vi "Get Teams.vi"(6 "Authorization":T2[](array[typedef]), 8 "error in (no error)":errorcluster) -> (0 "error out":errorcluster, 3 "Teams Out":T1(array[cluster]))   [LabVIEW 2016]
uses:
  <vilib>/addons/_JKI.lib/REST Client/classes/REST Client/HTTP Header.ctl
  <vilib>/addons/_JKI.lib/REST Client/classes/REST Client/REST Client.lvclass
  <vilib>/addons/_JKI.lib/Serialization/JSON/JKI JSON Serialization.lvlib
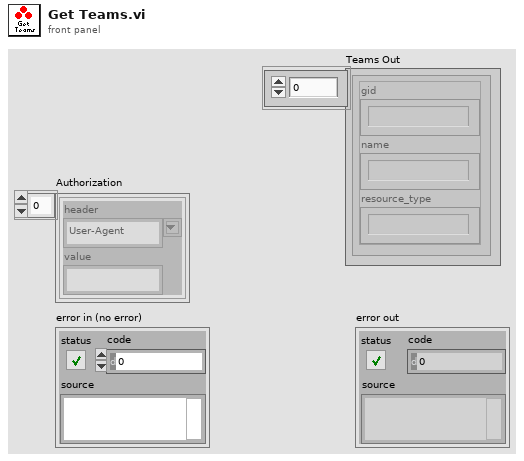
[diagram p1: front panel]
types:
  T1 = cluster{"gid":string, "name":string, "resource_type":string}[]
  T2 = typedef "REST Client.lvlib/REST Client.lvclass/HTTP Header.ctl" = cluster{"header":string, "value":string}
  T3 = cluster{"data":cluster{"gid":string, "name":string, "resource_type":string}[]}
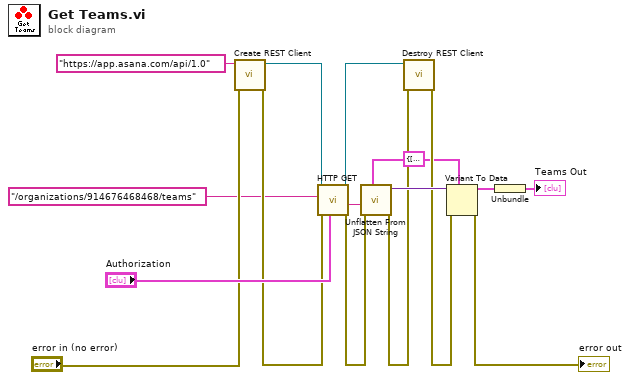
[diagram p0: block diagram]
diagram:
  w4 = T3 {"data"=[{"gid"="", "name"="", "resource_type"=""}, {"gid"="", "name"="", "resource_type"=""}]}
  n1 = call <vilib>:"Create REST Client.vi"("error in (no error)"="error in (no error)", "Base URL"="https://app.asana.com/api/1.0") -> ("error out"=w11:errorcluster, "REST Client out"=w14:refnum<class "REST Client.lvclass">)  [unwired: 8 in]
  n2 = call-dynamic "HTTP GET.vi"("request specific headers"="Authorization", "error in (no error)"=w11, "Path"="/organizations/914676468468/teams", "REST Client in"=w14) -> ("error out"=w8:errorcluster, "Response body"=w9:string, "REST Client out"=w13:refnum<class "REST Client.lvclass">)  [unwired: 2 in, 3 out]
  n3 = call <vilib>:"Unflatten From JSON String.vi"("Type and Defaults"=w4, "error in (no error)"=w8, "JSON String"=w9) -> ("error out"=w7:errorcluster, "Variant"=w10:variant)  [unwired: 7 in]
  n4 = call-dynamic "Destroy REST Client.vi"("error in (no error)"=w7, "REST Client in"=w13) -> ("error out"=w6:errorcluster)  [unwired: 9 in]
  n5 = Variant To Data(error in=w6, type=w4, Variant=w10) -> (data=w3:T3, error out=→"error out":errorcluster)
  n6 = Unbundle(w3) -> ("data"=→"Teams Out":T1)
